vi "practica1.vi"() -> ()   [LabVIEW 2018]
uses:
  <vilib>/imath/engines/lvmath/Plug In/_Char/NIMS_CH_character datatype.ctl
  <vilib>/imath/engines/lvmath2/RunTimeEngine/Managers/WorkSpace/UID Generator.vi
  <vilib>/imath/engines/lvmath2/RunTimeEngine/BuiltInFunctions/iir_butter/NIMS_[2o]_iir_butter(I32,V,Str).vi
  <vilib>/imath/engines/lvmath2/RunTimeEngine/ErrorHandling/NIMS_Create Error From Enums.vi
  <vilib>/imath/engines/lvmath2/RunTimeEngine/RunTimeType/NIMS_RunTimeType_From StrictType (excl LVString).vi
  <instcachedir>/0/NIMS_RunTimeType_From StrictType (excl LVString)_201635486D724C82825D35238731EDF5.lvgen/NIMS_RunTimeType_From StrictType (excl LVString)_201635486D724C82825D35238731EDF5_000.vi
  <vilib>/imath/engines/lvmath2/RunTimeEngine/LocalVariableDefStatement/MC_LocalVariableDefStatement_Display.vi
  <vilib>/imath/engines/lvmath2/RunTimeEngine/BuiltInFunctions/figure/NIMS_figure(I32).vi
  <vilib>/imathl/engines/lvmath/Functions/Error Handling/Create Error.vi
  <vilib>/imath/engines/lvmath2/RunTimeEngine/BuiltInFunctions/zplane/NIMS_zplane(M,M).vi
  <vilib>/imath/engines/lvmath2/RunTimeEngine/BuiltInFunctions/roots/NIMS_roots.vi
  <instcachedir>/0/NIMS_roots_5371068BAABD481CB00E0B78F1D2DC4F.lvgen/NIMS_roots_5371068BAABD481CB00E0B78F1D2DC4F_000.vi
  <vilib>/imath/engines/lvmath2/RunTimeEngine/ErrorHandling/NIMS_Error From Error Code.vi
  <vilib>/imath/engines/lvmath2/RunTimeSupport/NIMS_Complex To Real.vi
  <instcachedir>/0/NIMS_Complex To Real_355B64E31A464632BEBA00ACAE3499D9.lvgen/NIMS_Complex To Real_355B64E31A464632BEBA00ACAE3499D9_002.vi
  <vilib>/imath/engines/lvmath2/RunTimeEngine/BuiltInFunctions/filter_impulse/NIMS_filter_impulse.vi
  <vilib>/imath/engines/lvmath2/RunTimeEngine/BuiltInFunctions/freqzd/NIMS_freqzd().vi
  <vilib>/imath/engines/lvmath2/RunTimeEngine/BuiltInFunctions/hold/NIMS_hold(Enums).vi
  <vilib>/imath/engines/lvmath2/RunTimeEngine/BuiltInFunctions/abs/NIMS_abs(signed).vi
  <instcachedir>/0/NIMS_abs(signed)_C4FCB8E6058B49B797C7C8D53CA5F6EC.lvgen/NIMS_abs(signed)_C4FCB8E6058B49B797C7C8D53CA5F6EC_006.vi
  <vilib>/imath/engines/lvmath2/RunTimeEngine/BuiltInFunctions/plot/NIMS_plot(RM, RM, Str).vi
  <vilib>/imath/engines/lvmath2/RunTimeEngine/BuiltInFunctions/grid/NIMS_grid.vi
  <vilib>/imath/engines/lvmath/Plug In/_Char/NIMS_CH_Character RV to String.vi
  <vilib>/imath/engines/lvmath2/RunTimeEngine/BuiltInFunctions/xlabel/NIMS_xlabel.vi
  <vilib>/imath/engines/lvmath2/RunTimeEngine/BuiltInFunctions/title/NIMS_title.vi
  <vilib>/imath/engines/lvmath2/RunTimeEngine/Managers/SymbolTable/Clear UID.vi
  <vilib>/imath/engines/lvmath2/RunTimeEngine/ErrorHandling/NIMS_Finalize Error.vi
  <vilib>/imath/engines/lvmath2/RunTimeEngine/BuiltInFunctions/bilinear/NIMS_[V,V,S]=bilinear.vi
  <vilib>/imath/engines/lvmath2/RunTimeEngine/BuiltInFunctions/pause/NIMS_pause(S).vi
  <vilib>/imath/engines/lvmath2/RunTimeEngine/Managers/SymbolTable/NIMS_WorkSpace.lvlib
panel:
  in  "Fs":dbl
  in  "fc":dbl
  in  "-> Transformación bilineal\n <- Invarianza al impulso":bool
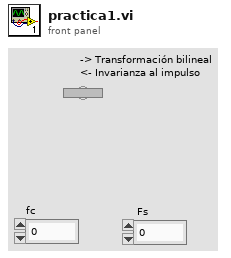
[diagram p1: front panel]
types:
  T1 = typedef "NIMS_CH_character datatype.ctl" = cluster{"Numeric":u8}
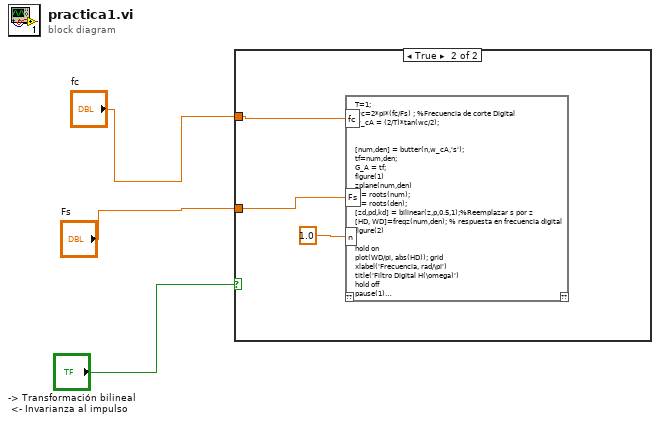
[diagram p0: block diagram]
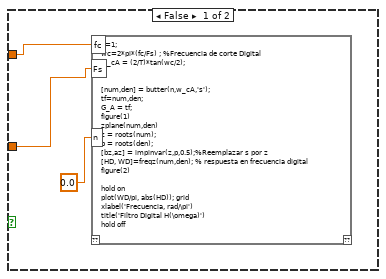
[diagram p2: hidden frame]
diagram:
  n1 = case shown="True" "-> Transformación bilineal\n <- Invarianza al impulso" {
    tunnel: "fc" -> [w4 w644]
    tunnel: "Fs" -> [w5 w645]
    frame False {
      n2 = mathscript code="T=1;\nwc=2*pi*(fc/Fs) ; %Frecuencia de corte Digital \nw_cA = (2/T)*tan(wc/2);\n\n\n[num,den] = butter(n,w_cA,'s');\ntf=num,den;\nG_A = tf;\nfigure(1)\nzplane(num,den)\nz = roots(num);\np = roots(den);\n[bz,az] = impinvar(z,p,0.5);%Reemplazar s por z\n[HD, WD]=freqz(num,den); % respuesta en frecuencia digital\nfigure(2) \n\nhold on\nplot(WD/pi, abs(HD)); grid\nxlabel('Frecuencia, rad/\\pi')\ntitle('Filtro Digital H(\\omega)')\nhold off\n\n\n\n\nT=1; \nwc=2*pi*(fc/Fs) ; %Frecuencia de corte Digital \nw_cA = (2/T)*tan(wc/2);\n\n\n[num,den] = butter(n,w_cA,'s');\ntf=num,den;\nG_A = tf;\nfigure(1)\nzplane(num,den)\nz = roots(num);\np = roots(den);\n[zd,pd] = impinvar(z,p,0.5);%Reemplazar s por z\n[HD, WD]=freqz(num,den); % respuesta en frecuencia digital\nfigure(2) \n\nhold on\nplot(WD/pi, abs(HD)); grid\nxlabel('Frecuencia, rad/\\pi')\ntitle('Filtro Digital H(\\omega)')\nhold off\n\n\nhold off"("fc"=w4, "Fs"=w5, "n"=0.0) -> ()  [unwired: 1 in, 1 out]
    }
    frame True {
      n3 = mathscript code="T=1; \nwc=2*pi*(fc/Fs) ; %Frecuencia de corte Digital \nw_cA = (2/T)*tan(wc/2);\n\n\n[num,den] = butter(n,w_cA,'s');\ntf=num,den;\nG_A = tf;\nfigure(1)\nzplane(num,den)\nz = roots(num);\np = roots(den);\n[zd,pd,kd] = bilinear(z,p,0.5,1);%Reemplazar s por z\n[HD, WD]=freqz(num,den); % respuesta en frecuencia digital\nfigure(2) \n\nhold on\nplot(WD/pi, abs(HD)); grid\nxlabel('Frecuencia, rad/\\pi')\ntitle('Filtro Digital H(\\omega)')\nhold off\npause(1)\n\nhold off"("fc"=w644, "Fs"=w645, "n"=1.0 ("input variable")) -> ()  [unwired: 1 in, 1 out]
    }
  }
